vi "AcquireSlowCtrl.vi"(7 "File Path":path=path "C:/Xe", 11 "LJConfig In":T2={"Negative Channels 2"=[3, 5, 7, 9, 199, 199, 199, 199, 199, 199, 199], "Positive Channels 2"=[2, 4, 6, 8, 0, 1, 10, 11, 12, 13, 14], "Handle Out"=0, "error out"={"status"=FALSE, "code"=0, "source"=""}, "IO Types Out"=[]}) -> (3 "Slow Control Data":T1)   [LabVIEW 2023]
uses:
  TypeDefs/DataTypes/LabJackConfig.ctl
  TypeDefs/DataTypes/SlowCtrlData.ctl
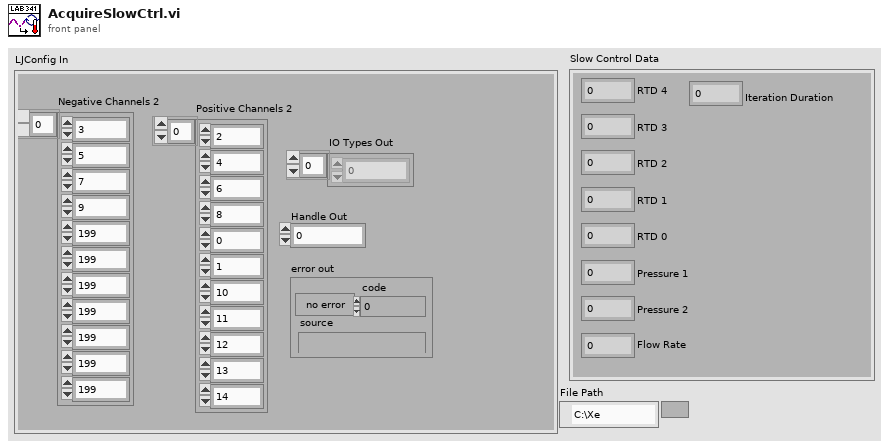
[diagram p1: front panel]
types:
  T1 = typedef "SlowCtrlData.ctl" = cluster{"RTD 0":dbl, "RTD 1":dbl, "RTD 2":dbl, "RTD 3":dbl, "RTD 4":dbl, "Pressure 1":dbl, "Pressure 2":dbl, "Flow Rate":dbl, "Iteration Duration":i64}
  T2 = typedef "LabJackConfig.ctl" = cluster{"Negative Channels 2":i32[], "Positive Channels 2":i32[], "Handle Out":i32, "error out":errorcluster, "IO Types Out":i32[]}
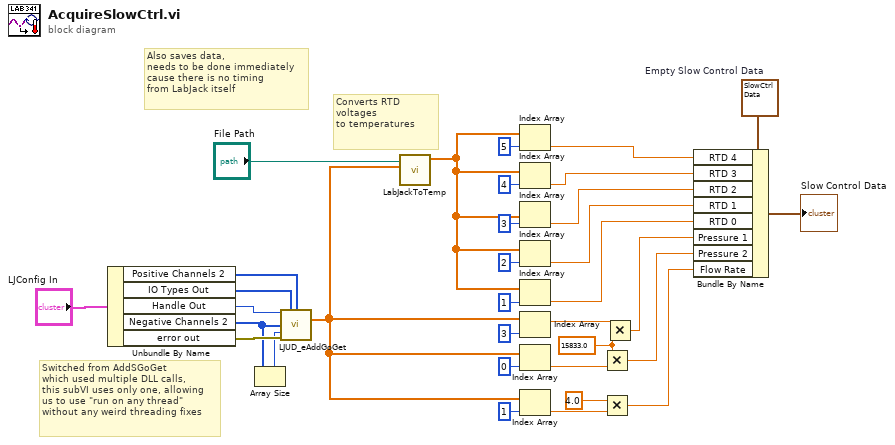
[diagram p0: block diagram]
diagram:
  w32 = T1 {"RTD 0"=0.0, "RTD 1"=0.0, "RTD 2"=0.0, "RTD 3"=0.0, "RTD 4"=0.0, "Pressure 1"=0.0, "Pressure 2"=0.0, "Flow Rate"=0.0, "Iteration Duration"=0}  # Empty Slow Control Data
  w21 = 15833.0 ("y")
  # "Also saves data,\nneeds to be done immediately\ncause there is no timing \nfrom LabJack itself"
  # "Switched from AddSGoGet\nwhich used multiple DLL calls,\nthis subVI uses only one, allowing\nus to use \"run on any thread\"\nwithout any weird threading fixes"
  # "Converts RTD voltages \nto temperatures"
  n1 = Unbundle By Name("LJConfig In") -> ("Positive Channels 2"=w8:i32[], "IO Types Out"=w7:i32[], "Handle Out"=w6:i32, "Negative Channels 2"=w4:i32[], "error out"=w5:errorcluster)
  n2 = Array Size(array=w4) -> (size(s)=w3:i32)
  n3 = call <vilib>:"LJUD_eAddGoGet.vi"("Handle In"=w6, "aIOTypes"=w7, "aChannels"=w8, "ax1s"=w4, "NumRequests"=w3, "error in"=w5) -> ("Values Read"=w2:dbl[])  [unwired: 4 in, 5 out]
  n4 = call "LabJackToTemp.vi"("LJ Data"=w2, "File Path"="File Path") -> ("Temperatures"=w18:dbl[])  [unwired: 9 in]
  n5 = Index Array(array=w18, index=5) -> (element=w23:dbl)
  n6 = Index Array(array=w18, index=4) -> (element=w33:dbl)
  n7 = Index Array(array=w18, index=3) -> (element=w24:dbl)
  n8 = Index Array(array=w18, index=2) -> (element=w25:dbl)
  n9 = Index Array(array=w18, index=1) -> (element=w26:dbl)
  n10 = Index Array(array=w2, index=3) -> (element=w22:dbl)
  n11 = Index Array(array=w2, index=0) -> (element=w15:dbl)
  n12 = Index Array(array=w2, index=1) -> (element=w19:dbl)
  n13 = Multiply(x=w21, y=w15) -> (x*y=w28:dbl)
  n14 = Multiply(x=4.0, y=w19) -> (x*y=w29:dbl)
  n15 = Multiply(x=w22, y=w21) -> (x*y=w27:dbl)
  n16 = Bundle By Name(cluster=w32, "RTD 4"=w23, "RTD 3"=w33, "RTD 2"=w24, "RTD 1"=w25, "RTD 0"=w26, "Pressure 1"=w27, "Pressure 2"=w28, "Flow Rate"=w29) -> (→"Slow Control Data":T1)
